vi "Close_loop_trajectory_Control_of_Tip.vi"() -> ()   [LabVIEW 2019]
uses:
  <vilib>/FPGAPlugInAG/sbRIO-9629/niLvFpga_Open_sbRIO-9629.vi
  <vilib>/rvi/interface/common/dynamic/niFpgaDynamicAddResources.vi
  <vilib>/Utility/error.llb/Error Cluster From Error Code.vi
  <vilib>/rvi/errors/niLvFpgaAdjustHostInterfaceError.vi
  <vilib>/FPGAPlugInAG/Dynamic/niLvFpga_Close_Dynamic.vi
  <vilib>/rvi/interface/nirviOpenFPGA/nirviOpenFPGA.xnode
  FPGA Bitfiles/fcmsinglesection_FPGATarget_CloseLoopMotorTu_eGt+d+EV+VE.lvbitx
  Close_Loop_Motor_Tune.vi
  <vilib>/rvi/interface/nirviReadWriteControl/nirviReadWriteControl.xnode
  <vilib>/rvi/interface/nirviCloseFPGA/nirviCloseFPGA.xnode
  NiFpgaLv.dll
  <vilib>/rvi/interface/Simulation/niFpgaSimulationCallBeginRW.vi
panel:
  in  "Motor3_KP":sgl
  in  "Motor2_KP":sgl
  in  "Motor1_KP":sgl
  out "Error":bool
  in  "Kp":dbl[](array[numeric])
  out "error":dbl[](array[numeric])
  out "Current Tip Coordinates":dbl[](array[numeric])
  out "data out":string
  out "Tip Position":dbl[](array[numeric])
  out "theta1":dbl
  out "theta2":dbl
  out "theta3":dbl
  out "L_v":dbl
  out "alpha":dbl
  in  "Time":dbl
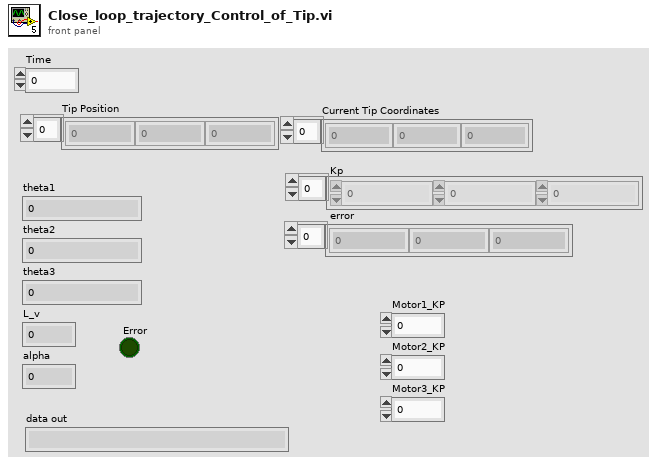
[diagram p1: front panel]
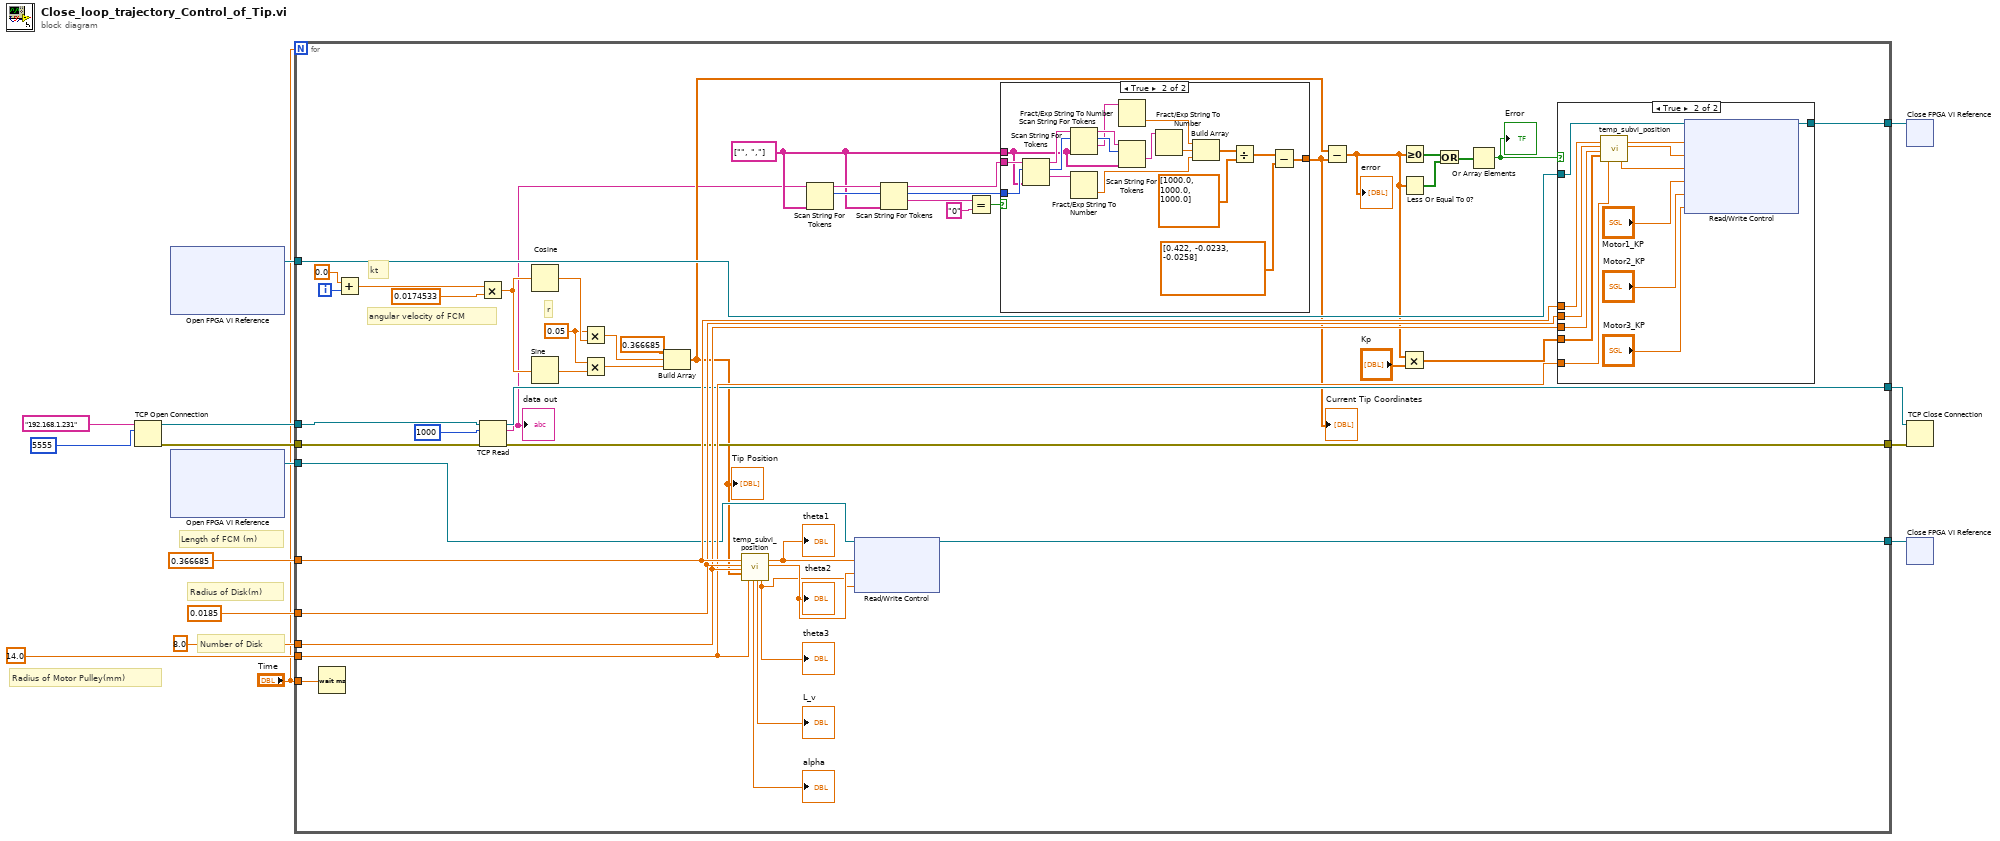
[diagram p0: block diagram]
diagram:
  # "Radius of Motor Pulley(mm)"
  # "Number of Disk"
  # "Radius of Disk(m)"
  # "Length of FCM (m)"
  n1 = TCP Open Connection(address="192.168.1.231", remote port or service name=u16 5555) -> (connection ID=w8:refnum<k5>, error out=w9:errorcluster)  [unwired: 3 in]
  n2 = xnode "Open FPGA VI Reference"() -> ("FPGA VI Reference Out"=w6:refnum<k20>)  [unwired: 2 in, 1 out]
  n3 = xnode "Open FPGA VI Reference"() -> ("FPGA VI Reference Out"=w5:refnum<k20>)  [unwired: 2 in, 1 out]
  n4 = for {
    N: "Time" -> [_]
    tunnel: "Time" -> [w57]
    tunnel: 0.366685 ("Length of the FCM (m)") -> [w61]
    tunnel: 0.0185 ("Radius of disk (m)") -> [w60]
    tunnel: 8.0 ("Number of Disks") -> [w59]
    tunnel: 14.0 ("Radius of motor pulley\n (mm)") -> [w58]
    tunnel: [w62] -> w10
    tunnel: w9 -> [w52]
    tunnel: w8 -> [w50]
    tunnel: w6 -> [w46]
    tunnel: w5 -> [w56]
    tunnel: [w49] -> w3
    tunnel: [w48] -> w2
    tunnel: [w47] -> w1
    i -> [w55]
    w28 = string[] ["", ","] ("delimiters (\\s,\\t,\\r,\\n)")
    w44 = 0.05
    # "angular velocity of FCM"
    # "r"
    # "kt"
    n5 = Wait (ms)(milliseconds to wait=w57) -> ()  [unwired: 1 out]
    n6 = Add(x=0.0, y=w55) -> (x+y=w53:dbl)
    n7 = Multiply(x=w53, y=0.0174533) -> (x*y=w40:dbl)
    n8 = TCP Read(connection ID=w50, bytes to read=1000, error in (no error)=w52) -> (connection ID out=w48:refnum<k5>, data out=w17:string, error out=w49:errorcluster)  [unwired: 2 in]
    "data out" <- w17
    n9 = Cosine(x=w40) -> (cos(x)=w45:dbl)
    n10 = Sine(x=w40) -> (sin(x)=w43:dbl)
    n11 = Multiply(x=w44, y=w45) -> (x*y=w42:dbl)
    n12 = Multiply(x=w44, y=w43) -> (x*y=w41:dbl)
    n13 = Build Array(0.366685, w42, w41) -> (w24:dbl[])
    "Tip Position" <- w24
    n14 = call "temp_subvi_position.vi"("Length of the FCM (m)"=w61, "Radius of disk (m)"=w60, "Number of Disks"=w59, "Tip position"=w24, "Radius of pulley (mm)"=w58) -> ("alpha"=→"alpha":dbl, "L_v"=→"L_v":dbl, "Theta 3"=w35:dbl, "Theta 1"=w37:dbl, "Theta 2"=w36:dbl)  [unwired: 4 in, 6 out]
    "theta1" <- w37
    "theta2" <- w36
    "theta3" <- w35
    n15 = Scan String For Tokens(6:w28, 9:w17) -> (2:w29:i32, 3:w30:string)  [unwired: 4 in, 2 out]
    n16 = xnode "Read/Write Control"("FPGA VI Reference In"=w56, "desired angle"=w37, "desired angle 2"=w36, "desired angle 3"=w35) -> ("FPGA VI Reference Out"=w62:refnum<k20>)  [unwired: 1 in, 1 out]
    n17 = Scan String For Tokens(6:w28, 8:w29, 9:w30) -> (1:w31:string, 2:w34:i32, 3:w33:string)  [unwired: 3 in, 1 out]
    n18 = Equal?(x=w31, y="0") -> (x = y?=w32:bool)
    n19 = case shown="True" w32 {
      tunnel: w33 -> [_ w90]
      tunnel: w34 -> [_ w89]
      tunnel: w28 -> [_ w88]
      tunnel: [_ w77] -> w26
      frame False {
      }
      frame True {
        n20 = Scan String For Tokens(6:w88, 8:w89, 9:w90) -> (1:w87:string, 2:w92:i32, 3:w94:string)  [unwired: 3 in, 1 out]
        n21 = Scan String For Tokens(6:w88, 8:w92, 9:w94) -> (1:w86:string, 2:w91:i32, 3:w93:string)  [unwired: 3 in, 1 out]
        n22 = Fract/Exp String To Number(string=w87) -> (number=w82:dbl)  [unwired: 3 in, 1 out]
        n23 = Fract/Exp String To Number(string=w86) -> (number=w84:dbl)  [unwired: 3 in, 1 out]
        n24 = Scan String For Tokens(6:w88, 8:w91, 9:w93) -> (1:w85:string)  [unwired: 3 in, 3 out]
        n25 = Fract/Exp String To Number(string=w85) -> (number=w83:dbl)  [unwired: 3 in, 1 out]
        n26 = Build Array(w84, w83, w82) -> (w81:dbl[])
        n27 = Divide(x=w81, y=dbl[] [1000.0, 1000.0, 1000.0]) -> (x/y=w79:dbl[])
        n28 = Subtract(x=w79, y=dbl[] [0.422, -0.0233, -0.0258]) -> (x-y=w77:dbl[])
      }
    }
    "Current Tip Coordinates" <- w26
    n29 = Subtract(x=w24, y=w26) -> (x-y=w23:dbl[])
    "error" <- w23
    n30 = Multiply(x=w23, y="Kp") -> (x*y=w18:dbl[])
    n31 = Greater Or Equal To 0?(x=w23) -> (x >= 0?=w22:bool[])
    n32 = Less Or Equal To 0?(x=w23) -> (x <= 0?=w21:bool[])
    n33 = Or(x=w22, y=w21) -> (x .or. y?=w20:bool[])
    n34 = Or Array Elements(Boolean array=w20) -> (logical OR=w19:bool)
    "Error" <- w19
    n35 = case shown="True" w19 {
      tunnel: w61 -> [_ w76]
      tunnel: w60 -> [_ w75]
      tunnel: w59 -> [_ w74]
      tunnel: w58 -> [_ w73]
      tunnel: w18 -> [_ w72]
      tunnel: [_ w71] -> w47
      tunnel: w46 -> [_ w67]
      frame False {
      }
      frame True {
        n36 = call "temp_subvi_position.vi"("Length of the FCM (m)"=w76, "Radius of disk (m)"=w75, "Number of Disks"=w74, "Tip position"=w72, "Radius of pulley (mm)"=w73) -> ("Theta 3"=w68:dbl, "Theta 1"=w69:dbl, "Theta 2"=w70:dbl)  [unwired: 4 in, 8 out]
        n37 = xnode "Read/Write Control"("FPGA VI Reference In"=w67, "desired angle (error)"=w69, "desired angle 2(error)"=w70, "desired angle 3(error)"=w68, "Motor1_KP"="Motor1_KP", "Motor2_KP"="Motor2_KP", "Motor3_KP"="Motor3_KP") -> ("FPGA VI Reference Out"=w71:refnum<k20>)  [unwired: 1 in, 1 out]
      }
    }
  }
  n38 = xnode "Close FPGA VI Reference"("FPGA VI Reference In"=w1) -> ()  [unwired: 1 in, 1 out]
  n39 = TCP Close Connection(connection ID=w2, error in (no error)=w3) -> ()  [unwired: 1 in, 2 out]
  n40 = xnode "Close FPGA VI Reference"("FPGA VI Reference In"=w10) -> ()  [unwired: 1 in, 1 out]
